vi "Periodic Tasks.vi"(8 "error in":errorcluster) -> ()   [LabVIEW 2012]
doc: "This VI runs in parallel to other tasks. It can contain as many user-defined periodic loops as you need. These can carry out PID or other sorts of timed response."
uses:
  <vilib>/Rock Robotics/SystemInterfaces/Utilities/FPGA_UtilitiesLED Source.ctl
  <vilib>/Rock Robotics/SystemInterfaces/Utilities/FPGA_UtilitiesLED State.ctl
  <vilib>/Rock Robotics/WPI/Solenoid/WPI_SolenoidValue.ctl
  <vilib>/Rock Robotics/WPI/Compressor/WPI_CompressorGetSetRefNum.vi
  Robot Global Data.vi
  <vilib>/Rock Robotics/WPI/Solenoid/WPI_SolenoidSetEnum.vi
  <vilib>/Rock Robotics/WPI/Joystick/WPI_JoystickGetSetRefNum.vi
  <vilib>/addons/control/pid/pid.llb/PID Advanced (DBL).vi
  <vilib>/addons/control/pid/NI_PID_pid.lvlib
panel:
  out "Aileron Error":dbl
  in  "linearity":dbl=0.5 format="%.2f"
  out "Shooter Speed":dbl(graph)
  out "Shooter Output":dbl
  in  "PID gains":T1={"proportional gain (Kc)"=0.002, "integral time (Ti, min)"=0.01, "derivative time (Td, min)"=0.001} {"derivative time (Td, min)" format="%#.5f"; "integral time (Ti, min)" format="%#.5f"; "proportional gain (Kc)" format="%#.5f"}
  out "Aileron Offset":dynamicdata(graph)
  out "Distance":dbl
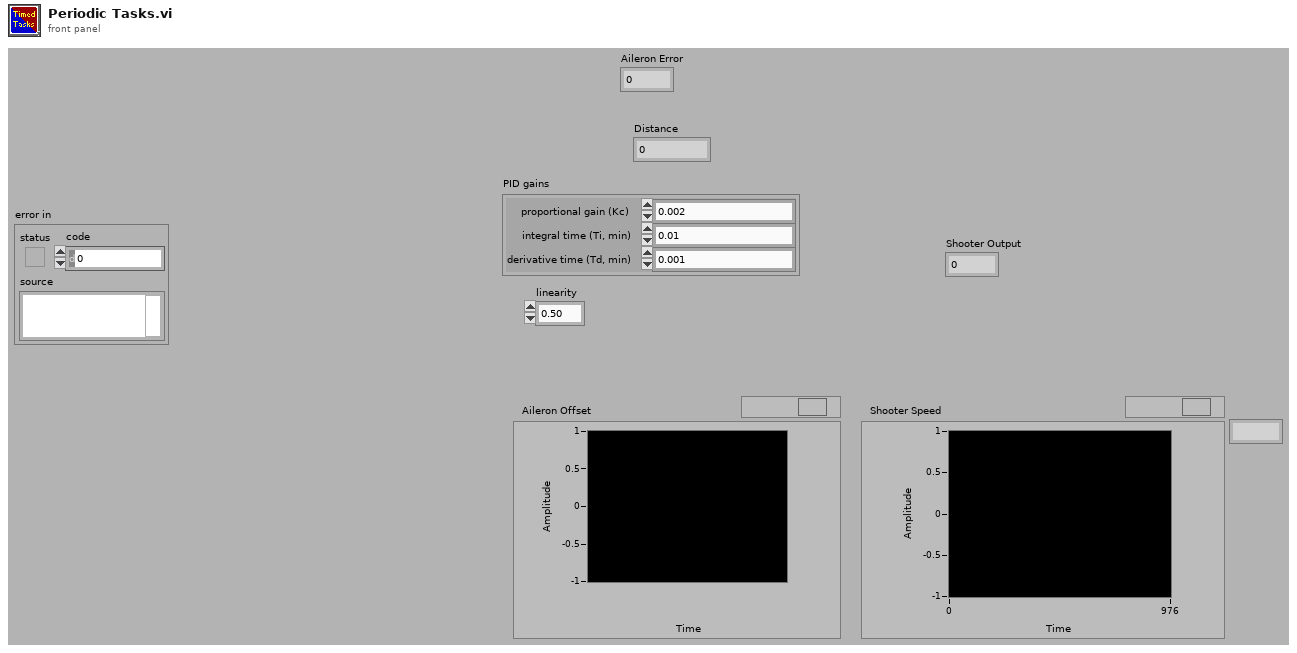
[diagram p1: front panel]
types:
  T1 = cluster{"proportional gain (Kc)":dbl, "integral time (Ti, min)":dbl, "derivative time (Td, min)":dbl}
  T2 = typedef "FPGA_UtilitiesLED State.ctl" = enum16{"Off", "On", "Toggle"}
  T3 = typedef "FPGA_UtilitiesLED Source.ctl" = enum16{"User LED", "FPGA LED"}
  T4 = typedef "WPI_SolenoidValue.ctl" = enum16{"Off", "On", "Forward", "Reverse"}
  T5 = typedef "WPI_SolenoidDevRef.ctl" = cluster{"DevStatus":errorcluster, "Solenoid Module":T6, "Forward Solenoid Channel":T7, "Reverse Solenoid Channel":T7}
  T6 = typedef "FPGA_TypedefSolenoidModule.ctl" = enum16{"Solenoid Module 1", "Solenoid Module 2"}
  T7 = typedef "WPI_SolenoidChannel.ctl" = enum8{"Solenoid 1", "Solenoid 2", "Solenoid 3", "Solenoid 4", "Solenoid 5", "Solenoid 6", "Solenoid 7", "Solenoid 8", "Invalid"}
  T8 = typedef "WPI_DigitalInputDevRef.ctl" = cluster{"DevStatus":errorcluster, "DIO Channel":T9, "Digital Module":T10}
  T9 = typedef "FPGA_DIOChannel.ctl" = enum8{"DIO 1", "DIO 2", "DIO 3", "DIO 4", "DIO 5", "DIO 6", "DIO 7", "DIO 8", "DIO 9", "DIO 10", "DIO 11", "DIO 12", "DIO 13", "DIO 14", "Invalid"}
  T10 = typedef "FPGA_TypedefDigitalModule.ctl" = enum16{"Digital Module 1", "Digital Module 2"}
  T11 = typedef "WPI_MotorControlDeviceRef.ctl" = cluster{"DeviceStatus":errorcluster, "Type":enum16{"PWM", "CAN"}, "PWM":cluster{"Digital Module":T10, "PWM Channel":T12, "DeadBand":T13}, "CAN":cluster{"Device Number":u8, "Control Mode":T14, "Semaphore":T15, "Max Vout":dbl}, "Invert":bool, "TransformRef":T16, "InvTransformRef":T16}
  T12 = typedef "FPGA_DIOPWMChannel.ctl" = enum8{"PWM 1", "PWM 2", "PWM 3", "PWM 4", "PWM 5", "PWM 6", "PWM 7", "PWM 8", "PWM 9", "PWM 10", "Invalid"}
  T13 = typedef "WPI_PWMDeadband.ctl" = cluster{"Name":string, "maxPositivePwm":i32, "minPositivePwm":i32, "centerPwm":i32, "maxNegativePwm":i32, "minNegativePwm":i32, "angularRange":u16}
  T14 = typedef "WPI_CANJaguar_ControlMode.ctl" = enum8{"Percent VBus", "Current", "Speed", "Position", "Voltage"}
  T15 = typedef "Semaphore RefNum" = refnum<k1>
  T16 = typedef "WPI_PWMTransform_ConPane.ctl" = refnum<vi>
  T17 = typedef "WPI_CounterDevRef.ctl" = cluster{"DevStatus":errorcluster, "CntIndex":T18}
  T18 = typedef "FPGA_CounterCtrSystemIndex.ctl" = enum8{"Ctr 0", "Ctr 1", "Ctr 2", "Ctr 3", "Ctr 4", "Ctr 5", "Ctr 6", "Ctr 7", "Invalid"}
  T19 = typedef "WPI_CompressorDevRef.ctl" = cluster{"DevStatus":errorcluster, "DigitalInputDevRef":T8, "RelayDevRef":T20}
  T20 = typedef "WPI_RelayDevRef.ctl" = cluster{"DevStatus":errorcluster, "Relay Channel":T21, "Digital Module":T10, "Relay Direction":T22}
  T21 = typedef "FPGA_DIORelayChannel.ctl" = enum8{"Relay 1", "Relay 2", "Relay 3", "Relay 4", "Relay 5", "Relay 6", "Relay 7", "Relay 8", "Invalid"}
  T22 = typedef "WPI_RelayDirection.ctl" = enum16{"Both directions", "Forward only", "Reverse only"}
  T23 = typedef "WPI_EncoderDevRef.ctl" = cluster{"DevStatus":errorcluster, "EncoderIndex":T24, "CounterIndex":T18, "DistancePerCount":dbl, "Decoding Type":T25}
  T24 = typedef "FPGA_EncoderIdx.ctl" = enum8{"Enc 0", "Enc 1", "Enc 2", "Enc 3", "Invalid"}
  T25 = typedef "WPI_EncoderType.ctl" = enum16{"1x", "2x", "4x"}
  T26 = enum16{"Standard", "Buffered", "CRLF", "Immediate"}
  T27 = typedef "WPI_JoystickDevRef.ctl" = cluster{"Device":T28}
  T28 = typedef "WPI_JoystickDeviceEnum.ctl" = enum16{"USB 1", "USB 2", "USB 3", "USB 4", "Kinect 1", "Kinect 2"}
  T29 = typedef "WPI_JoystickButtonState.ctl" = cluster{"Button 1":bool, "Button 2":bool, "Button 3":bool, "Button 4":bool, "Button 5":bool, "Button 6":bool, "Button 7":bool, "Button 8":bool, "Button 9":bool, "Button 10":bool, "Button 11":bool, "Button 12":bool}
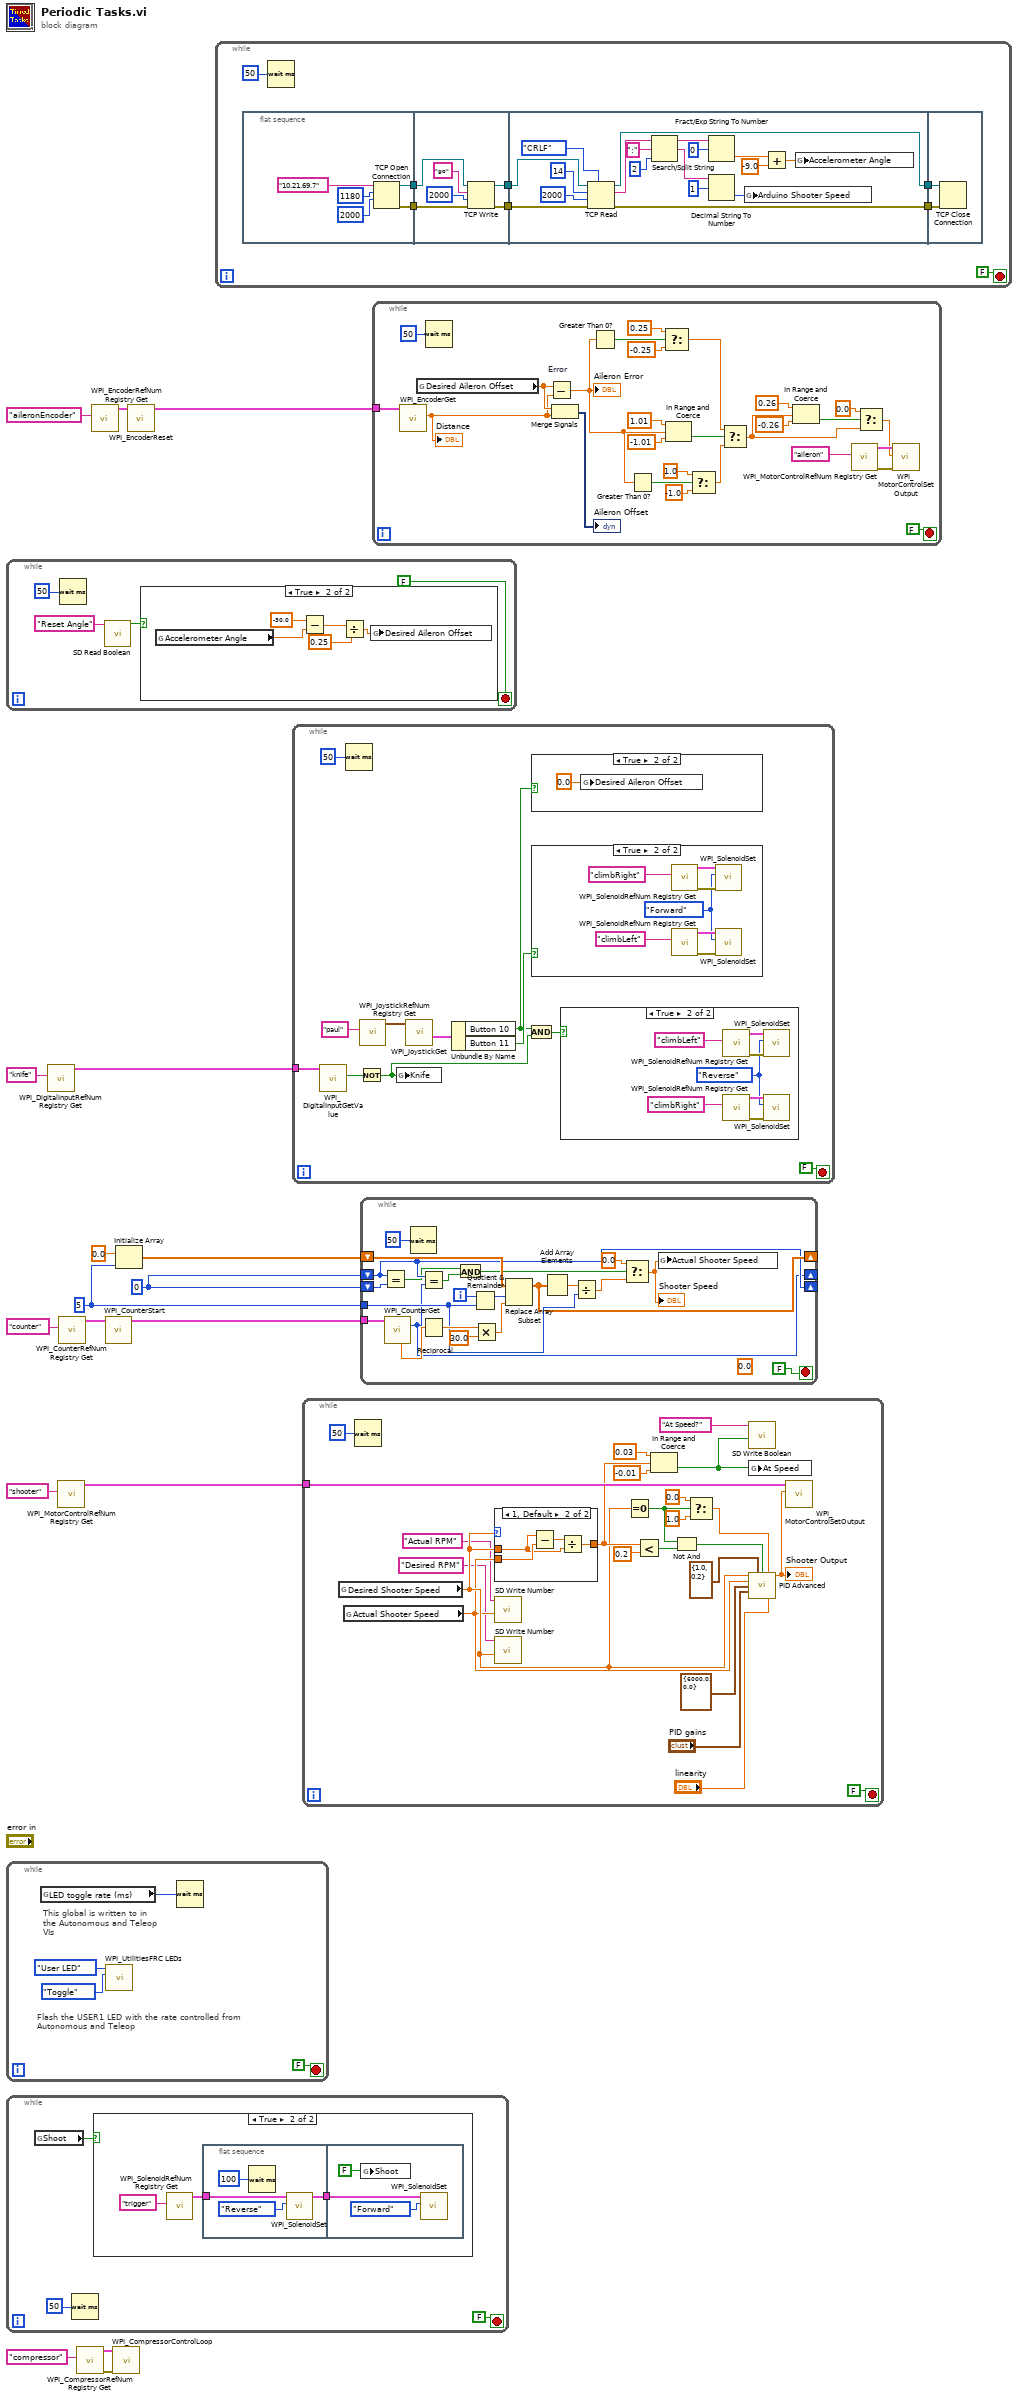
[diagram p0: block diagram]
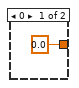
[diagram p7: hidden frame]
diagram:
  w1 = 0
  w4 = 5 ("dimension size")
  n1 = while {
    stop <- FALSE stop-if-true
    n2 = Wait (ms)(milliseconds to wait=u32 50) -> ()  [unwired: 1 out]
    n3 = call <vilib>:"SD Read Boolean.vi"("Name"="Reset Angle") -> ("Boolean"=w19:bool)  [unwired: 8 in, 2 out]
    n4 = case shown="True" w19 {
      frame False {
      }
      frame True {
        n5 = global read "Robot Global Data.vi" "Accelerometer Angle"() -> (w26:dbl)
        n6 = Subtract(x=-30.0, y=w26) -> (x-y=w24:dbl)
        n7 = Divide(x=w24, y=0.25) -> (x/y=w22:dbl)
        n8 = global write "Robot Global Data.vi" "Desired Aileron Offset"(w22) -> ()
      }
    }
  }
  n9 = while {
    stop <- FALSE stop-if-true
    # "This global is written to in the Autonomous and Teleop VIs"
    # "Flash the USER1 LED with the rate controlled from Autonomous and Teleop"
    n10 = global read "Robot Global Data.vi" "LED toggle rate (ms)"() -> (w27:u32)
    n11 = call <vilib>:"WPI_UtilitiesFRC LEDs.vi"("State"=FPGA_UtilitiesLED_State."Toggle", "LED Type"=FPGA_UtilitiesLED_Source."User LED") -> ()  [unwired: 1 in, 9 out]
    n12 = Wait (ms)(milliseconds to wait=w27) -> ()  [unwired: 1 out]
  }
  n13 = while {
    stop <- FALSE stop-if-true
    n14 = global read "Robot Global Data.vi" "Shoot"() -> (w31:bool)
    n15 = Wait (ms)(milliseconds to wait=u32 50) -> ()  [unwired: 1 out]
    n16 = case shown="True" w31 {
      frame False {
      }
      frame True {
        n17 = call <vilib>:"WPI_SolenoidRefNum Registry Get.vi"("refnum name"="trigger") -> ("SolenoidDevRef"=w34:T5)  [unwired: 9 in, 1 out]
        n18 = flat-sequence {
          tunnel: w34 -> [w38]
          tunnel: [w37] -> w36
          tunnel: w36 -> [w42]
          frame #0 {
            n19 = Wait (ms)(milliseconds to wait=u32 100) -> ()  [unwired: 1 out]
            n20 = call-poly <vilib>:"WPI_SolenoidSet.vi"("Value"=WPI_SolenoidValue."Reverse", "SolenoidDevRef"=w38) -> ("SolenoidDevRef"=w37:T5)  [unwired: 8 in, 1 out]
          }
          frame #1 {
            n21 = global write "Robot Global Data.vi" "Shoot"(FALSE) -> ()
            n22 = call-poly <vilib>:"WPI_SolenoidSet.vi"("Value"=WPI_SolenoidValue."Forward", "SolenoidDevRef"=w42) -> ()  [unwired: 8 in, 2 out]
          }
        }
      }
    }
  }
  n23 = call <vilib>:"WPI_DigitalInputRefNum Registry Get.vi"("refnum name"="knife") -> ("DigitalInputDevRef"=w3:T8)  [unwired: 9 in, 1 out]
  n24 = call <vilib>:"WPI_MotorControlRefNum Registry Get.vi"("refnum name"="shooter") -> ("MotorControlDevRef"=w8:T11)  [unwired: 9 in, 1 out]
  n25 = call <vilib>:"WPI_CounterRefNum Registry Get.vi"("refnum name"="counter") -> ("CounterDevRef"=w10:T17)  [unwired: 9 in, 1 out]
  n26 = call <vilib>:"WPI_CompressorRefNum Registry Get.vi"("refnum name"="compressor") -> ("error out"=w12:errorcluster, "CompressorDevRef"=w14:T19)  [unwired: 9 in]
  n27 = call <vilib>:"WPI_EncoderRefNum Registry Get.vi"("refnum name"="aileronEncoder") -> ("EncoderDevRef"=w15:T23)  [unwired: 9 in, 1 out]
  n28 = call <vilib>:"WPI_CounterStart.vi"("CounterDevRef in"=w10) -> ("CounterDevRef out"=w11:T17)  [unwired: 9 in, 1 out]
  n29 = call <vilib>:"WPI_CompressorControlLoop.vi"("error in (no error)"=w12, "CompressorDevRef"=w14) -> ()  [unwired: 10 in]
  n30 = Initialize Array(0.0 ("element"), w4) -> (w5:dbl[])
  n31 = call <vilib>:"WPI_EncoderReset.vi"("EncoderDevRef"=w15) -> ("EncoderDevRef"=w16:T23)  [unwired: 9 in, 1 out]
  n32 = while {
    stop <- FALSE stop-if-true
    n33 = flat-sequence {
      tunnel: [w53] -> w51
      tunnel: [w52] -> w50
      tunnel: w51 -> [w62]
      tunnel: w50 -> [w61]
      tunnel: [w58] -> w49
      tunnel: [w57] -> w48
      tunnel: w49 -> [w80]
      tunnel: w48 -> [w79]
      tunnel: [w75] -> w47
      tunnel: [w74] -> w46
      tunnel: w47 -> [w82]
      tunnel: w46 -> [w81]
      frame #0 {
        n34 = TCP Open Connection(address="10.21.69.7", remote port or service name=u16 1180, timeout ms (60000)=2000) -> (connection ID=w53:refnum<k5>, error out=w52:errorcluster)  [unwired: 2 in]
      }
      frame #1 {
        n35 = TCP Write(connection ID=w62, data in="go", error in (no error)=w61, 9:2000 ("timeout ms (25000)")) -> (connection ID out=w57:refnum<k5>, error out=w58:errorcluster)  [unwired: 1 out]
      }
      frame #2 {
        n36 = TCP Read(connection ID=w79, bytes to read=14, error in (no error)=w80, 7:T26."CRLF" ("mode (standard)"), 9:2000 ("timeout ms (25000)")) -> (connection ID out=w74:refnum<k5>, data out=w72:string, error out=w75:errorcluster)
        n37 = Search/Split String(string=w72, search string/char (-)=":", offset (0)=2) -> (substring before match=w70:string, match + rest of string=w67:string)  [unwired: 1 out]
        n38 = Fract/Exp String To Number(string=w70, offset=0) -> (number=w65:dbl)  [unwired: 2 in, 1 out]
        n39 = Decimal String To Number(string=w67, offset=1) -> (number=w66:i32)  [unwired: 1 in, 1 out]
        n40 = global write "Robot Global Data.vi" "Arduino Shooter Speed"(w66) -> ()
        n41 = Add(x=w65, y=-9.0) -> (x+y=w64:dbl)
        n42 = global write "Robot Global Data.vi" "Accelerometer Angle"(w64) -> ()
      }
      frame #3 {
        n43 = TCP Close Connection(connection ID=w81, error in (no error)=w82) -> ()  [unwired: 1 in, 2 out]
      }
    }
    n44 = Wait (ms)(milliseconds to wait=u32 50) -> ()  [unwired: 1 out]
  }
  n45 = while {
    tunnel: w3 -> [w93]
    stop <- FALSE stop-if-true
    n46 = call <vilib>:"WPI_DigitalInputGetValue.vi"("DigitalInputDevRef"=w93) -> ("Value"=w92:bool)  [unwired: 8 in, 2 out]
    n47 = Wait (ms)(milliseconds to wait=u32 50) -> ()  [unwired: 1 out]
    n48 = Not(x=w92) -> (.not. x?=w87:bool)
    n49 = call <vilib>:"WPI_JoystickRefNum Registry Get.vi"("refnum name"="paul") -> ("JoystickDevRef"=w89:T27)  [unwired: 9 in, 1 out]
    n50 = global write "Robot Global Data.vi" "Knife"(w87) -> ()
    n51 = call <vilib>:"WPI_JoystickGet.vi"("JoystickDevRef"=w89) -> ("Buttons"=w88:T29)  [unwired: 4 in, 2 out]
    n52 = Unbundle By Name(w88) -> ("Button 10"=w83:bool, "Button 11"=w84:bool)
    n53 = And(x=w83, y=w87) -> (x .and. y?=w86:bool)
    n54 = case shown="True" w83 {
      frame False {
      }
      frame True {
        n55 = global write "Robot Global Data.vi" "Desired Aileron Offset"(0.0 ("Desired Aileron Offset")) -> ()
      }
    }
    n56 = case shown="True" w84 {
      frame False {
      }
      frame True {
        w97 = WPI_SolenoidValue."Forward" ("Value")
        n57 = call <vilib>:"WPI_SolenoidRefNum Registry Get.vi"("refnum name"="climbRight") -> ("error out"=w100:errorcluster, "SolenoidDevRef"=w101:T5)  [unwired: 9 in]
        n58 = call <vilib>:"WPI_SolenoidRefNum Registry Get.vi"("refnum name"="climbLeft") -> ("error out"=w99:errorcluster, "SolenoidDevRef"=w98:T5)  [unwired: 9 in]
        n59 = call-poly <vilib>:"WPI_SolenoidSet.vi"("error in (no error)"=w100, "Value"=w97, "SolenoidDevRef"=w101) -> ()  [unwired: 7 in, 2 out]
        n60 = call-poly <vilib>:"WPI_SolenoidSet.vi"("error in (no error)"=w99, "Value"=w97, "SolenoidDevRef"=w98) -> ()  [unwired: 7 in, 2 out]
      }
    }
    n61 = case shown="True" w86 {
      frame False {
      }
      frame True {
        w104 = WPI_SolenoidValue."Reverse" ("Value")
        n62 = call <vilib>:"WPI_SolenoidRefNum Registry Get.vi"("refnum name"="climbLeft") -> ("error out"=w106:errorcluster, "SolenoidDevRef"=w105:T5)  [unwired: 9 in]
        n63 = call <vilib>:"WPI_SolenoidRefNum Registry Get.vi"("refnum name"="climbRight") -> ("error out"=w107:errorcluster, "SolenoidDevRef"=w108:T5)  [unwired: 9 in]
        n64 = call-poly <vilib>:"WPI_SolenoidSet.vi"("error in (no error)"=w106, "Value"=w104, "SolenoidDevRef"=w105) -> ()  [unwired: 7 in, 2 out]
        n65 = call-poly <vilib>:"WPI_SolenoidSet.vi"("error in (no error)"=w107, "Value"=w104, "SolenoidDevRef"=w108) -> ()  [unwired: 7 in, 2 out]
      }
    }
  }
  n66 = while {
    tunnel: w8 -> [w130]
    stop <- FALSE stop-if-true
    n67 = global read "Robot Global Data.vi" "Desired Shooter Speed"() -> (w112:dbl)
    n68 = global read "Robot Global Data.vi" "Actual Shooter Speed"() -> (w111:dbl)
    n69 = Wait (ms)(milliseconds to wait=u32 50) -> ()  [unwired: 1 out]
    n70 = case shown="1, Default" w112 {
      tunnel: [0.0 w137] -> w117
      tunnel: w111 -> [_ w136]
      tunnel: w112 -> [_ w135]
      frame 0 {
      }
      frame 1, Default {
        n71 = Subtract(x=w135, y=w136) -> (x-y=w134:dbl)
        n72 = Divide(x=w134, y=w135) -> (x/y=w137:dbl)
      }
    }
    n73 = call <vilib>:"SD Write Number.vi"("Numeric"=w111, "Name"="Actual RPM") -> ()  [unwired: 8 in, 2 out]
    n74 = call <vilib>:"SD Write Number.vi"("Numeric"=w112, "Name"="Desired RPM") -> ()  [unwired: 8 in, 2 out]
    n75 = Equal To 0?(x=w112) -> (x = 0?=w119:bool)
    n76 = Less?(x=w117, y=0.2) -> (x < y?=w120:bool)
    n77 = In Range and Coerce(upper limit=0.03, x=w117, lower limit=-0.01) -> (In Range?=w114:bool)  [unwired: 1 out]
    n78 = Not And(1:w120, 2:w119) -> (0:w118:bool)
    n79 = Select(t=0.0, s=w119, f=1.0) -> (s? t:f=w125:dbl)
    n80 = call <vilib>:"SD Write Boolean.vi"("Boolean"=w114, "Name"="At Speed?") -> ()  [unwired: 8 in, 2 out]
    n81 = global write "Robot Global Data.vi" "At Speed"(w114) -> ()
    n82 = call-poly <vilib>:"PID Advanced.vi"("setpoint"=w112, "output range"=cluster{"output high":dbl, "output low":dbl} {"output high"=1.0, "output low"=0.2}, "auto? (T)"=w118, "manual control"=w125, "process variable"=w111, "setpoint range"=cluster{"setpoint high":dbl, "setpoint low":dbl} {"setpoint high"=6000.0, "setpoint low"=0.0}, "PID gains"="PID gains", "linearity"="linearity") -> ("output"=w121:dbl)  [unwired: 6 in, 1 out]
    "Shooter Output" <- w121
    n83 = call <vilib>:"WPI_MotorControlSetOutput.vi"("Output"=w121, "MotorControlDevRef"=w130) -> ()  [unwired: 7 in, 3 out]
  }
  n84 = while {
    tunnel: w11 -> [w157]
    tunnel: w4 -> [w149]
    shift-right: [w147] -> _
    shift-left: w5 -> [w152]
    shift-right: [w141] -> _
    shift-left: w1 -> [w142]
    shift-right: [w142] -> _
    shift-left: w1 -> [w143]
    i -> [w150]
    stop <- FALSE stop-if-true
    (unwired) 0.0 ("t")
    n85 = Equal?(x=w142, y=w143) -> (x = y?=w140:bool)
    n86 = call <vilib>:"WPI_CounterGet.vi"("CounterDevRef in"=w157) -> ("Value"=w141:i32, "Period (sec)"=w156:dbl)  [unwired: 5 in, 4 out]
    n87 = Wait (ms)(milliseconds to wait=u32 50) -> ()  [unwired: 1 out]
    n88 = Equal?(x=w142, y=w141) -> (x = y?=w139:bool)
    n89 = Reciprocal(x=w156) -> (1/x=w155:dbl)
    n90 = And(x=w140, y=w139) -> (x .and. y?=w138:bool)
    n91 = Quotient & Remainder(x=w150, y=w149) -> (x-y*floor(x/y)=w148:i32)  [unwired: 1 out]
    n92 = Multiply(x=w155, y=30.0) -> (x*y=w151:dbl)
    n93 = Replace Array Subset(array=w152, new element=w151, index=w148) -> (w147:dbl[])
    n94 = Add Array Elements(numeric array=w147) -> (sum=w153:dbl)
    n95 = Divide(x=w153, y=w149) -> (x/y=w145:dbl)
    n96 = Select(t=0.0, s=w138, f=w145) -> (s? t:f=w144:dbl)
    "Shooter Speed" <- w144
    n97 = global write "Robot Global Data.vi" "Actual Shooter Speed"(w144) -> ()
  }
  n98 = while {
    tunnel: w16 -> [w181]
    stop <- FALSE stop-if-true
    n99 = call <vilib>:"WPI_EncoderGet.vi"("EncoderDevRef"=w181) -> ("Distance"=w178:dbl)  [unwired: 5 in, 5 out]
    "Distance" <- w178
    n100 = global read "Robot Global Data.vi" "Desired Aileron Offset"() -> (w179:dbl)
    n101 = Wait (ms)(milliseconds to wait=u32 50) -> ()  [unwired: 1 out]
    n102 = Subtract "Error"(x=w179, y=w178) -> (x-y=w160:dbl)
    "Aileron Error" <- w160
    n103 = Merge Signals(w179, w178) -> (→"Aileron Offset":dynamicdata)
    n104 = Greater Than 0?(x=w160) -> (x > 0?=w161:bool)
    n105 = Greater Than 0?(x=w160) -> (x > 0?=w177:bool)
    n106 = Select(t=0.25, s=w161, f=-0.25) -> (s? t:f=w168:dbl)
    n107 = In Range and Coerce(upper limit=1.01 ("lower limit"), x=w160, lower limit=-1.01) -> (In Range?=w171:bool)  [unwired: 1 out]
    n108 = Select(t=1.0, s=w177, f=-1.0) -> (s? t:f=w176:dbl)
    n109 = Select(t=w168, s=w171, f=w176) -> (s? t:f=w163:dbl)
    n110 = In Range and Coerce(upper limit=0.26 ("lower limit"), x=w163, lower limit=-0.26) -> (In Range?=w165:bool)  [unwired: 1 out]
    n111 = call <vilib>:"WPI_MotorControlRefNum Registry Get.vi"("refnum name"="aileron") -> ("error out"=w182:errorcluster, "MotorControlDevRef"=w183:T11)  [unwired: 9 in]
    n112 = Select(t=0.0, s=w165, f=w163) -> (s? t:f=w162:dbl)
    n113 = call <vilib>:"WPI_MotorControlSetOutput.vi"("error in (no error)"=w182, "Output"=w162, "MotorControlDevRef"=w183) -> ()  [unwired: 6 in, 3 out]
  }
